vi "Ploymorphic Mean.vi"   [LabVIEW 2014]
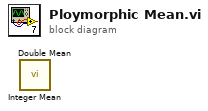
[diagram p0: block diagram]
diagram:
  n1 = call "Integer Mean.vi"() -> ()  [unwired: 11 in, 1 out]
  n2 = call "Double Mean.vi"() -> ()  [unwired: 11 in, 1 out]
